vi "Teleop.vi"(10 "Match Info":T1={"Autonomous Elapsed Seconds"=0.0, "TeleOp Elapsed Seconds"=0.0, "Disabled Elapsed Seconds"=0.0, "Visited Autonomous"=FALSE, "Visited TeleOp"=FALSE, "Visited Disabled"=FALSE, "Autonomous Settings"={"Autonomous Style"=enum."Independent", "VI Refnum"=refnum}}, 11 "Call Context":T2) -> ()   [LabVIEW 2012]
doc: "This VI is called for each TeleOp packet received from the DS where the robot is not disabled. It is often used to read from the joysticks and update I/O or to update setpoints for timed control loops. It should complete and return within 20 milliseconds or it may miss DS packets."
uses:
  <vilib>/Rock Robotics/WPI/DriverStation/WPI_DriverStationDerivedRobotMode.ctl
  <vilib>/Rock Robotics/WPI/DriverStation/WPI_DriverStationMatch Info.ctl
  <vilib>/Rock Robotics/WPI/Relay/WPI_RelayValue.ctl
  Robot Global Data.vi
  <vilib>/Rock Robotics/WPI/Joystick/WPI_JoystickGetSetRefNum.vi
panel:
  in  "PTO Disabled":dbl=90.0
  in  "PTO Enabled":dbl=140.0
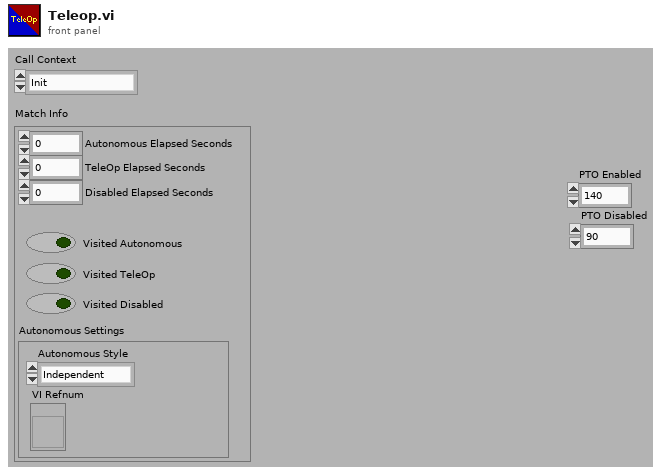
[diagram p1: front panel]
types:
  T1 = typedef "WPI_DriverStationMatch Info.ctl" = cluster{"Autonomous Elapsed Seconds":dbl, "TeleOp Elapsed Seconds":dbl, "Disabled Elapsed Seconds":dbl, "Visited Autonomous":bool, "Visited TeleOp":bool, "Visited Disabled":bool, "Autonomous Settings":cluster{"Autonomous Style":enum16{"Iterative", "Independent"}, "VI Refnum":refnum<vi>}}
  T2 = typedef "WPI_DriverStationDerivedRobotMode.ctl" = enum16{"Init", "Execute", "Stop"}
  T3 = typedef "WPI_RelayValue.ctl" = enum16{"Off", "On", "Forward", "Reverse"}
  T4 = typedef "WPI_MotorControlDeviceRef.ctl" = cluster{"DeviceStatus":errorcluster, "Type":enum16{"PWM", "CAN"}, "PWM":cluster{"Digital Module":T5, "PWM Channel":T6, "DeadBand":T7}, "CAN":cluster{"Device Number":u8, "Control Mode":T8, "Semaphore":T9, "Max Vout":dbl}, "Invert":bool, "TransformRef":T10, "InvTransformRef":T10}
  T5 = typedef "FPGA_TypedefDigitalModule.ctl" = enum16{"Digital Module 1", "Digital Module 2"}
  T6 = typedef "FPGA_DIOPWMChannel.ctl" = enum8{"PWM 1", "PWM 2", "PWM 3", "PWM 4", "PWM 5", "PWM 6", "PWM 7", "PWM 8", "PWM 9", "PWM 10", "Invalid"}
  T7 = typedef "WPI_PWMDeadband.ctl" = cluster{"Name":string, "maxPositivePwm":i32, "minPositivePwm":i32, "centerPwm":i32, "maxNegativePwm":i32, "minNegativePwm":i32, "angularRange":u16}
  T8 = typedef "WPI_CANJaguar_ControlMode.ctl" = enum8{"Percent VBus", "Current", "Speed", "Position", "Voltage"}
  T9 = typedef "Semaphore RefNum" = refnum<k1>
  T10 = typedef "WPI_PWMTransform_ConPane.ctl" = refnum<vi>
  T11 = cluster{"Driver Station Digital Input (1-8)[0]":bool, "Driver Station Digital Input (1-8)[1]":bool, "Driver Station Digital Input (1-8)[2]":bool, "Driver Station Digital Input (1-8)[3]":bool, "Driver Station Digital Input (1-8)[4]":bool, "Driver Station Digital Input (1-8)[5]":bool, "Driver Station Digital Input (1-8)[6]":bool, "Driver Station Digital Input (1-8)[7]":bool, "Driver Station Digital Input (1-8)[8]":bool}
  T12 = typedef "WPI_JoystickDevRef.ctl" = cluster{"Device":T13}
  T13 = typedef "WPI_JoystickDeviceEnum.ctl" = enum16{"USB 1", "USB 2", "USB 3", "USB 4", "Kinect 1", "Kinect 2"}
  T14 = cluster{"axis 1 (x)":dbl, "axis 2 (y)":dbl, "axis 3 (throttle)":dbl, "axis 4":dbl, "axis 5":dbl, "axis 6":dbl}
  T15 = typedef "WPI_ServoDeviceRef.ctl" = cluster{"DeviceStatus":errorcluster, "Digital Module":T5, "PWM Channel":T6, "DeadBand":T7}
  T16 = typedef "WPI_RelayDevRef.ctl" = cluster{"DevStatus":errorcluster, "Relay Channel":T17, "Digital Module":T5, "Relay Direction":T18}
  T17 = typedef "FPGA_DIORelayChannel.ctl" = enum8{"Relay 1", "Relay 2", "Relay 3", "Relay 4", "Relay 5", "Relay 6", "Relay 7", "Relay 8", "Invalid"}
  T18 = typedef "WPI_RelayDirection.ctl" = enum16{"Both directions", "Forward only", "Reverse only"}
  T19 = typedef "WPI_JoystickButtonState.ctl" = cluster{"Button 1":bool, "Button 2":bool, "Button 3":bool, "Button 4":bool, "Button 5":bool, "Button 6":bool, "Button 7":bool, "Button 8":bool, "Button 9":bool, "Button 10":bool, "Button 11":bool, "Button 12":bool}
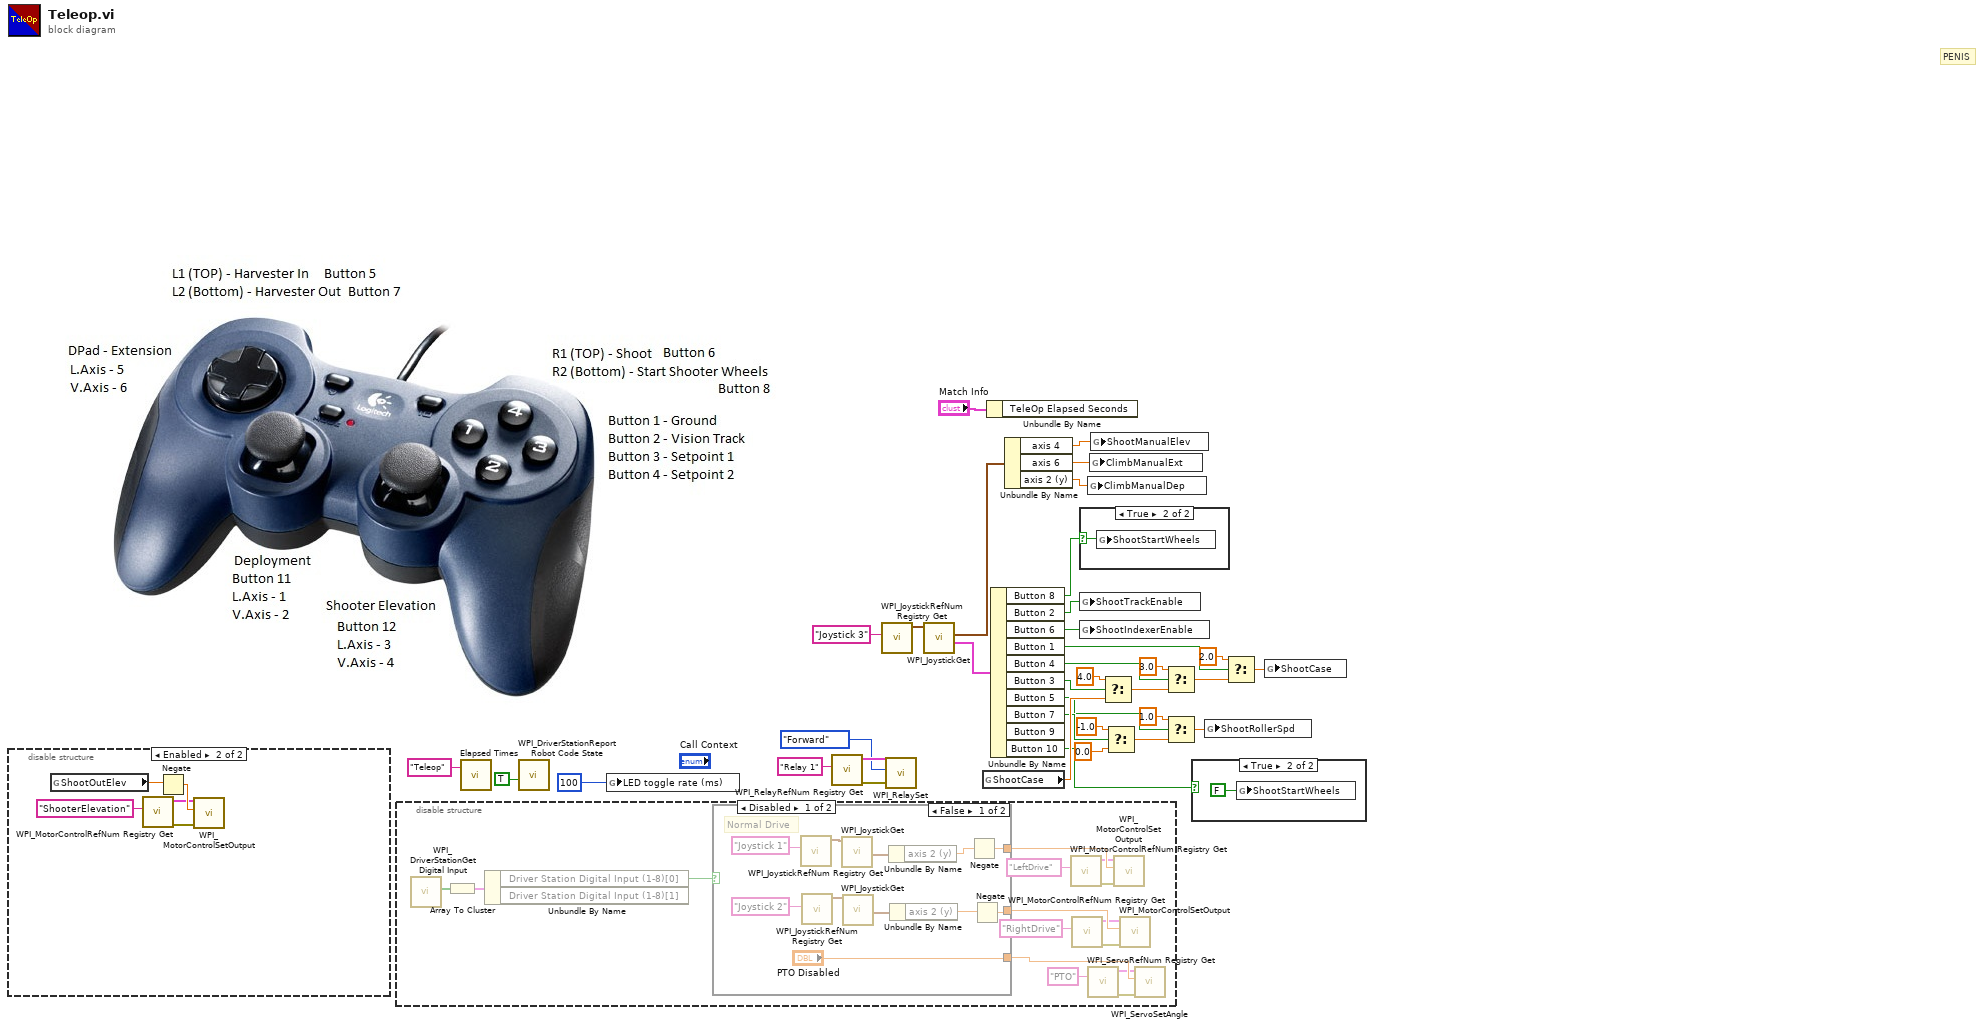
[diagram p0: block diagram]
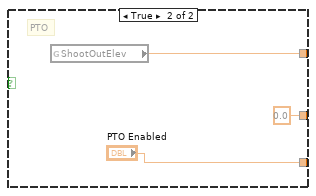
[diagram p2: hidden frame]
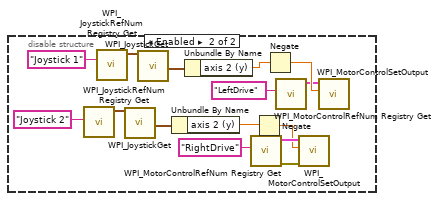
[diagram p3: hidden frame]
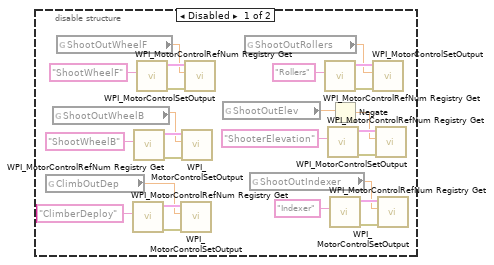
[diagram p4: hidden frame]
diagram:
  # "PENIS"
  n1 = disable-structure shown="Enabled" {
    frame Disabled {
      n2 = global read "Robot Global Data.vi" "ClimbOutDep"() -> (w37:dbl)
      n3 = global read "Robot Global Data.vi" "ShootOutWheelB"() -> (w38:dbl)
      n4 = global read "Robot Global Data.vi" "ShootOutWheelF"() -> (w43:dbl)
      n5 = call <vilib>:"WPI_MotorControlRefNum Registry Get.vi"("refnum name"="ClimberDeploy") -> ("error out"=w55:errorcluster, "MotorControlDevRef"=w54:T4)  [unwired: 9 in]
      n6 = call <vilib>:"WPI_MotorControlRefNum Registry Get.vi"("refnum name"="ShootWheelB") -> ("error out"=w56:errorcluster, "MotorControlDevRef"=w57:T4)  [unwired: 9 in]
      n7 = call <vilib>:"WPI_MotorControlRefNum Registry Get.vi"("refnum name"="ShootWheelF") -> ("error out"=w61:errorcluster, "MotorControlDevRef"=w60:T4)  [unwired: 9 in]
      n8 = call <vilib>:"WPI_MotorControlSetOutput.vi"("error in (no error)"=w55, "Output"=w37, "MotorControlDevRef"=w54) -> ()  [unwired: 6 in, 3 out]
      n9 = call <vilib>:"WPI_MotorControlSetOutput.vi"("error in (no error)"=w56, "Output"=w38, "MotorControlDevRef"=w57) -> ()  [unwired: 6 in, 3 out]
      n10 = call <vilib>:"WPI_MotorControlSetOutput.vi"("error in (no error)"=w61, "Output"=w43, "MotorControlDevRef"=w60) -> ()  [unwired: 6 in, 3 out]
      n11 = global read "Robot Global Data.vi" "ShootOutElev"() -> (w40:dbl)
      n12 = global read "Robot Global Data.vi" "ShootOutRollers"() -> (w41:dbl)
      n13 = global read "Robot Global Data.vi" "ShootOutIndexer"() -> (w42:dbl)
      n14 = call <vilib>:"WPI_MotorControlRefNum Registry Get.vi"("refnum name"="Rollers") -> ("error out"=w50:errorcluster, "MotorControlDevRef"=w51:T4)  [unwired: 9 in]
      n15 = call <vilib>:"WPI_MotorControlRefNum Registry Get.vi"("refnum name"="ShooterElevation") -> ("error out"=w49:errorcluster, "MotorControlDevRef"=w48:T4)  [unwired: 9 in]
      n16 = Negate(x=w40) -> (-x=w39:dbl)
      n17 = call <vilib>:"WPI_MotorControlRefNum Registry Get.vi"("refnum name"="Indexer") -> ("error out"=w44:errorcluster, "MotorControlDevRef"=w45:T4)  [unwired: 9 in]
      n18 = call <vilib>:"WPI_MotorControlSetOutput.vi"("error in (no error)"=w50, "Output"=w41, "MotorControlDevRef"=w51) -> ()  [unwired: 6 in, 3 out]
      n19 = call <vilib>:"WPI_MotorControlSetOutput.vi"("error in (no error)"=w49, "Output"=w39, "MotorControlDevRef"=w48) -> ()  [unwired: 6 in, 3 out]
      n20 = call <vilib>:"WPI_MotorControlSetOutput.vi"("error in (no error)"=w44, "Output"=w42, "MotorControlDevRef"=w45) -> ()  [unwired: 6 in, 3 out]
    }
    frame Enabled {
      n21 = global read "Robot Global Data.vi" "ShootOutElev"() -> (w65:dbl)
      n22 = call <vilib>:"WPI_MotorControlRefNum Registry Get.vi"("refnum name"="ShooterElevation") -> ("error out"=w62:errorcluster, "MotorControlDevRef"=w63:T4)  [unwired: 9 in]
      n23 = Negate(x=w65) -> (-x=w66:dbl)
      n24 = call <vilib>:"WPI_MotorControlSetOutput.vi"("error in (no error)"=w62, "Output"=w66, "MotorControlDevRef"=w63) -> ()  [unwired: 6 in, 3 out]
    }
  }
  n25 = disable-structure shown="Disabled" {
    frame Disabled {
      n26 = call <vilib>:"WPI_DriverStationGet Digital Input.vi"() -> ("Driver Station Digital Input (1-8)"=w81:bool[])  [unwired: 11 in]
      n27 = Array To Cluster(array=w81) -> (cluster=w80:T11)
      n28 = Unbundle By Name(w80) -> ("Driver Station Digital Input (1-8)[0]"=w79:bool)  [unwired: 1 out]
      n29 = case shown="False" w79 {
        tunnel: [w84 w94] -> w76
        tunnel: [w83 0.0] -> w73
        tunnel: ["PTO Disabled" "PTO Enabled"] -> w70
        frame False {
          # "Normal Drive"
          n30 = call <vilib>:"WPI_JoystickRefNum Registry Get.vi"("refnum name"="Joystick 1") -> ("JoystickDevRef"=w86:T12)  [unwired: 1 in, 9 out]
          n31 = call <vilib>:"WPI_JoystickRefNum Registry Get.vi"("refnum name"="Joystick 2") -> ("JoystickDevRef"=w89:T12)  [unwired: 1 in, 9 out]
          n32 = call <vilib>:"WPI_JoystickGet.vi"("JoystickDevRef"=w86) -> ("Axes"=w87:T14)  [unwired: 1 in, 5 out]
          n33 = call <vilib>:"WPI_JoystickGet.vi"("JoystickDevRef"=w89) -> ("Axes"=w88:T14)  [unwired: 1 in, 5 out]
          n34 = Unbundle By Name(w87) -> ("axis 2 (y)"=w92:dbl)
          n35 = Unbundle By Name(w88) -> ("axis 2 (y)"=w91:dbl)
          n36 = Negate(x=w92) -> (-x=w84:dbl)
          n37 = Negate(x=w91) -> (-x=w83:dbl)
        }
        frame True {
          # "PTO"
          n38 = global read "Robot Global Data.vi" "ShootOutElev"() -> (w94:dbl)
        }
      }
      n39 = call <vilib>:"WPI_MotorControlRefNum Registry Get.vi"("refnum name"="LeftDrive") -> ("error out"=w74:errorcluster, "MotorControlDevRef"=w75:T4)  [unwired: 9 in]
      n40 = call <vilib>:"WPI_MotorControlRefNum Registry Get.vi"("refnum name"="RightDrive") -> ("error out"=w71:errorcluster, "MotorControlDevRef"=w72:T4)  [unwired: 9 in]
      n41 = call <vilib>:"WPI_ServoRefNum Registry Get.vi"("refnum name"="PTO") -> ("error out"=w69:errorcluster, "ServoDeviceRef"=w68:T15)  [unwired: 9 in]
      n42 = call <vilib>:"WPI_MotorControlSetOutput.vi"("error in (no error)"=w74, "Output"=w76, "MotorControlDevRef"=w75) -> ()  [unwired: 6 in, 3 out]
      n43 = call <vilib>:"WPI_MotorControlSetOutput.vi"("error in (no error)"=w71, "Output"=w73, "MotorControlDevRef"=w72) -> ()  [unwired: 6 in, 3 out]
      n44 = call <vilib>:"WPI_ServoSetAngle.vi"("error in (no error)"=w69, "Angle"=w70, "ServoDeviceRef"=w68) -> ()  [unwired: 7 in, 2 out]
    }
    frame Enabled {
      n45 = call <vilib>:"WPI_JoystickRefNum Registry Get.vi"("refnum name"="Joystick 2") -> ("JoystickDevRef"=w104:T12)  [unwired: 1 in, 9 out]
      n46 = call <vilib>:"WPI_JoystickRefNum Registry Get.vi"("refnum name"="Joystick 1") -> ("JoystickDevRef"=w102:T12)  [unwired: 1 in, 9 out]
      n47 = call <vilib>:"WPI_JoystickGet.vi"("JoystickDevRef"=w104) -> ("Axes"=w103:T14)  [unwired: 1 in, 5 out]
      n48 = call <vilib>:"WPI_JoystickGet.vi"("JoystickDevRef"=w102) -> ("Axes"=w96:T14)  [unwired: 1 in, 5 out]
      n49 = Unbundle By Name(w103) -> ("axis 2 (y)"=w106:dbl)
      n50 = Unbundle By Name(w96) -> ("axis 2 (y)"=w97:dbl)
      n51 = call <vilib>:"WPI_MotorControlRefNum Registry Get.vi"("refnum name"="RightDrive") -> ("error out"=w107:errorcluster, "MotorControlDevRef"=w110:T4)  [unwired: 9 in]
      n52 = Negate(x=w106) -> (-x=w109:dbl)
      n53 = Negate(x=w97) -> (-x=w100:dbl)
      n54 = call <vilib>:"WPI_MotorControlRefNum Registry Get.vi"("refnum name"="LeftDrive") -> ("MotorControlDevRef"=w98:T4)  [unwired: 9 in, 1 out]
      n55 = call <vilib>:"WPI_MotorControlSetOutput.vi"("error in (no error)"=w107, "Output"=w109, "MotorControlDevRef"=w110) -> ()  [unwired: 6 in, 3 out]
      n56 = call <vilib>:"WPI_MotorControlSetOutput.vi"("Output"=w100, "MotorControlDevRef"=w98) -> ()  [unwired: 7 in, 3 out]
    }
  }
  n57 = call "Elapsed Times.vi"("Call Name"="Teleop") -> ()  [unwired: 2 in, 1 out]
  n58 = call <vilib>:"WPI_DriverStationReport Robot Code State.vi"("TeleOp"=TRUE ("Autonomous")) -> ()  [unwired: 10 in, 1 out]
  n59 = global write "Robot Global Data.vi" "LED toggle rate (ms)"(u32 100 ("LED ms toggle rate")) -> ()
  n60 = call <vilib>:"WPI_RelayRefNum Registry Get.vi"("refnum name"="Relay 1") -> ("error out"=w31:errorcluster, "RelayDevRef"=w33:T16)  [unwired: 9 in]
  n61 = call <vilib>:"WPI_JoystickRefNum Registry Get.vi"("refnum name"="Joystick 3") -> ("JoystickDevRef"=w29:T12)  [unwired: 9 in, 1 out]
  n62 = call <vilib>:"WPI_RelaySet.vi"("error in (no error)"=w31, "RelayValue"=WPI_RelayValue."Forward", "RelayDevRef"=w33) -> ()  [unwired: 7 in, 2 out]
  n63 = call <vilib>:"WPI_JoystickGet.vi"("JoystickDevRef"=w29) -> ("Buttons"=w27:T19, "Axes"=w26:T14)  [unwired: 4 in, 1 out]
  n64 = global read "Robot Global Data.vi" "ShootCase"() -> (w13:dbl)
  n65 = Unbundle By Name("Match Info") -> ()  [unwired: 1 out]
  n66 = Unbundle By Name(w27) -> ("Button 8"=w4:bool, "Button 2"=w24:bool, "Button 6"=w25:bool, "Button 1"=w21:bool, "Button 4"=w19:bool, "Button 3"=w18:bool, "Button 5"=w9:bool, "Button 7"=w11:bool, "Button 10"=w3:bool)  [unwired: 1 out]
  n67 = Unbundle By Name(w26) -> ("axis 4"=w23:dbl, "axis 6"=w22:dbl, "axis 2 (y)"=w2:dbl)
  n68 = case shown="True" w4 {
    selector: w4 -> [_ w111]
    frame False {
    }
    frame True {
      n69 = global write "Robot Global Data.vi" "ShootStartWheels"(w111) -> ()
    }
  }
  n70 = global write "Robot Global Data.vi" "ShootTrackEnable"(w24) -> ()
  n71 = global write "Robot Global Data.vi" "ShootIndexerEnable"(w25) -> ()
  n72 = global write "Robot Global Data.vi" "ClimbManualDep"(w2) -> ()
  n73 = global write "Robot Global Data.vi" "ClimbManualExt"(w22) -> ()
  n74 = global write "Robot Global Data.vi" "ShootManualElev"(w23) -> ()
  n75 = Select(t=4.0, s=w18, f=w13) -> (s? t:f=w17:dbl)
  n76 = Select(t=-1.0, s=w11, f=0.0) -> (s? t:f=w10:dbl)
  n77 = Select(t=3.0, s=w19, f=w17) -> (s? t:f=w15:dbl)
  n78 = Select(t=1.0, s=w9, f=w10) -> (s? t:f=w5:dbl)
  n79 = case shown="True" w3 {
    frame False {
    }
    frame True {
      n80 = global write "Robot Global Data.vi" "ShootStartWheels"(FALSE ("ShootStartWheels")) -> ()
    }
  }
  n81 = global write "Robot Global Data.vi" "ShootRollerSpd"(w5) -> ()
  n82 = Select(t=2.0, s=w21, f=w15) -> (s? t:f=w12:dbl)
  n83 = global write "Robot Global Data.vi" "ShootCase"(w12) -> ()
